vi "create.AddOrderLong.vi"(8 "error in (no error)":errorcluster, 10 "AddOrder.Parms":T1, 11 "AddOrderLong in":refnum<class "AddOrderLong.lvclass">) -> (0 "error out":errorcluster, 3 "AddOrderLong out":refnum<class "AddOrderLong.lvclass">)   [LabVIEW 2022 SP3, in "AddOrderLong.lvclass"]
uses:
  AddOrderLong.lvclass
  FieldSpec.ctl
  PitchMessage/FieldValue.ctl
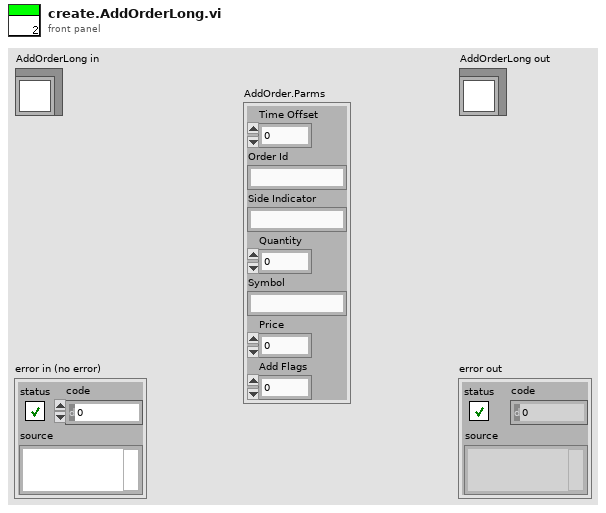
[diagram p1: front panel]
types:
  T1 = cluster{"Time Offset":u32, "Order Id":string, "Side Indicator":string, "Quantity":u32, "Symbol":string, "Price":dbl, "Add Flags":u8}
  T2 = typedef "FieldSpec.ctl" = cluster{"Name":string, "Offset":i32, "Length":i32, "FieldType":enum16{"Alphanumeric", "Binary", "BinaryLongPrice", "BinaryShortPrice", "BitField", "PrintableAscii", "Value"}}
  T3 = typedef "FieldValue.ctl" = variant
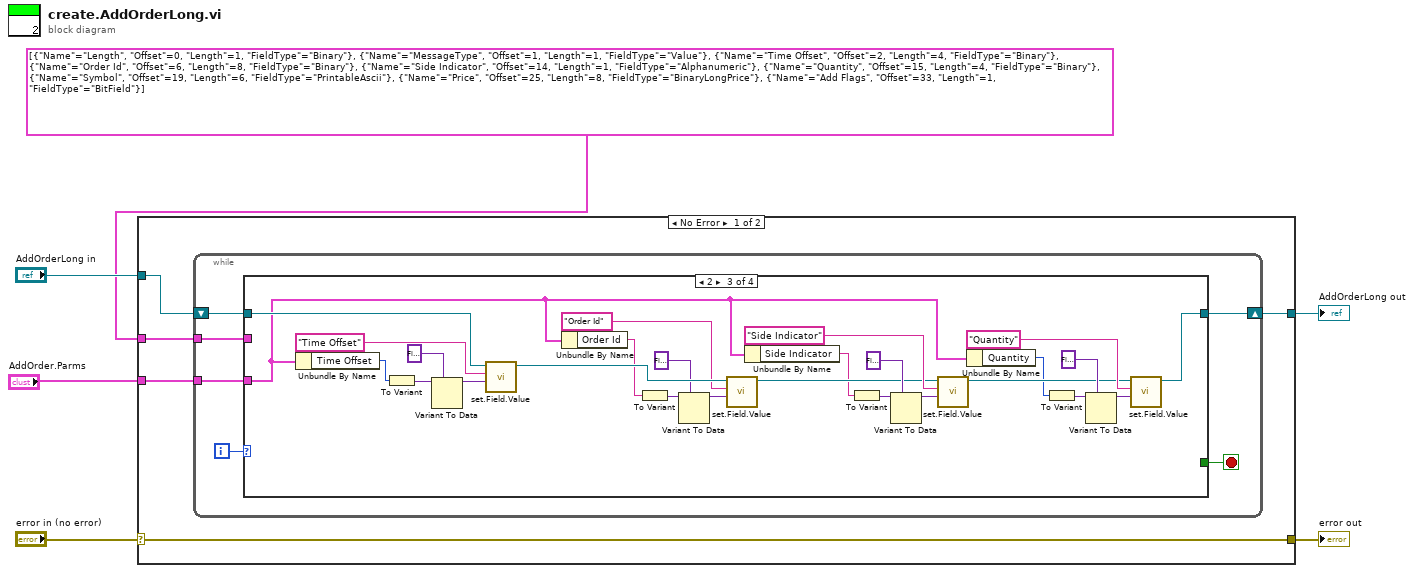
[diagram p0: block diagram]
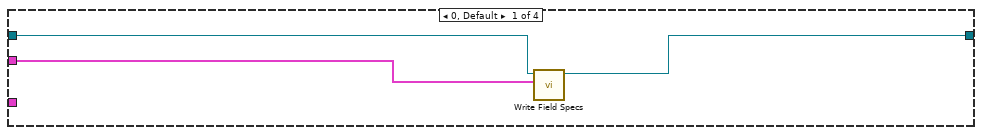
[diagram p2: hidden frame]
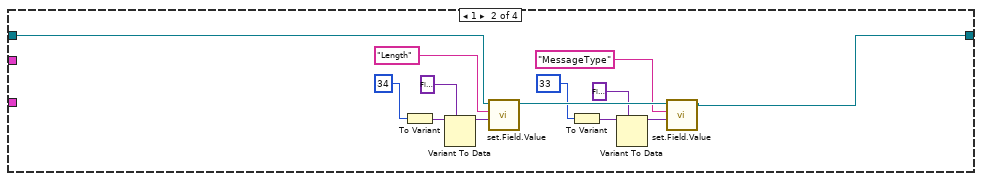
[diagram p3: hidden frame]
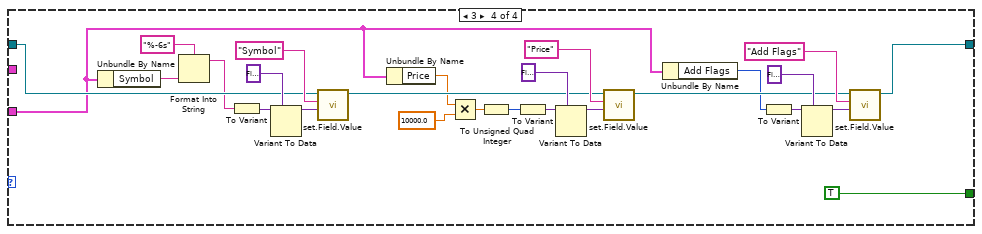
[diagram p4: hidden frame]
diagram:
  n1 = case shown="No Error" "error in (no error)" {
    selector: "error in (no error)" -> [w11 w87]
    tunnel: [w11 w87] -> w5
    tunnel: [w8 w86] -> w3
    tunnel: "AddOrderLong in" -> [w9 w86]
    tunnel: T2[] [{"Name"="Length", "Offset"=0, "Length"=1, "FieldType"=enum."Binary"}, {"Name"="MessageType", "Offset"=1, "Length"=1, "FieldType"=enum."Value"}, {"Name"="Time Offset", "Offset"=2, "Length"=4, "FieldType"=enum."Binary"}, {"Name"="Order Id", "Offset"=6, "Length"=8, "FieldType"=enum."Binary"}, {"Name"="Side Indicator", "Offset"=14, "Length"=1, "FieldType"=enum."Alphanumeric"}, {"Name"="Quantity", "Offset"=15, "Length"=4, "FieldType"=enum."Binary"}, {"Name"="Symbol", "Offset"=19, "Length"=6, "FieldType"=enum."PrintableAscii"}, {"Name"="Price", "Offset"=25, "Length"=8, "FieldType"=enum."BinaryLongPrice"}, {"Name"="Add Flags", "Offset"=33, "Length"=1, "FieldType"=enum."BitField"}] ("appended array") -> [w10 _]
    tunnel: "AddOrder.Parms" -> [w7 _]
    frame No Error {
      n2 = while {
        tunnel: w10 -> [w16]
        shift-right: [w14] -> w8
        shift-left: w9 -> [w15]
        tunnel: w7 -> [w12]
        i -> [w17]
        stop <- w13 stop-if-true
        n3 = case shown="2" w17 {
          tunnel: [_ _ _ TRUE] -> w13
          tunnel: w16 -> [w20 _ _ _]
          tunnel: w15 -> [w19 w22 w50 w81]
          tunnel: [w18 w21 w39 w64] -> w14
          tunnel: w12 -> [_ _ w35 w61]
          frame 0, Default {
            n4 = call-dynamic "Write Field Specs.vi"("Field Specs"=w20, "PitchMessage in"=w19) -> ("PitchMessage out"=w18:refnum<class "AddOrderLong.lvclass">)  [unwired: 8 in, 1 out]
          }
          frame 1 {
            n5 = To Variant(anything=u8 34 ("Value")) -> (Variant=w29:variant)
            n6 = Variant To Data(type=T3 variant ("FieldValue"), Variant=w29) -> (data=w30:T3)  [unwired: 1 in, 1 out]
            n7 = call-dynamic "set.Field.Value.vi"("Value"=w30, "FIeld.Name"="Length", "PitchMessage in"=w22) -> ("PitchMessage out"=w31:refnum<class "AddOrderLong.lvclass">)  [unwired: 7 in, 1 out]
            n8 = To Variant(anything=u8 33 ("Value")) -> (Variant=w32:variant)
            n9 = Variant To Data(type=T3 variant ("FieldValue"), Variant=w32) -> (data=w33:T3)  [unwired: 1 in, 1 out]
            n10 = call-dynamic "set.Field.Value.vi"("Value"=w33, "FIeld.Name"="MessageType", "PitchMessage in"=w31) -> ("PitchMessage out"=w21:refnum<class "AddOrderLong.lvclass">)  [unwired: 7 in, 1 out]
          }
          frame 2 {
            n11 = Unbundle By Name(w35) -> ("Time Offset"=w38:u32)
            n12 = To Variant(anything=w38) -> (Variant=w55:variant)
            n13 = Variant To Data(type=T3 variant ("FieldValue"), Variant=w55) -> (data=w56:T3)  [unwired: 1 in, 1 out]
            n14 = call-dynamic "set.Field.Value.vi"("Value"=w56, "FIeld.Name"="Time Offset", "PitchMessage in"=w50) -> ("PitchMessage out"=w58:refnum<class "AddOrderLong.lvclass">)  [unwired: 7 in, 1 out]
            n15 = Unbundle By Name(w35) -> ("Order Id"=w37:string)
            n16 = To Variant(anything=w37) -> (Variant=w57:variant)
            n17 = Variant To Data(type=T3 variant ("FieldValue"), Variant=w57) -> (data=w59:T3)  [unwired: 1 in, 1 out]
            n18 = call-dynamic "set.Field.Value.vi"("Value"=w59, "FIeld.Name"="Order Id", "PitchMessage in"=w58) -> ("PitchMessage out"=w45:refnum<class "AddOrderLong.lvclass">)  [unwired: 7 in, 1 out]
            n19 = Unbundle By Name(w35) -> ("Side Indicator"=w36:string)
            n20 = To Variant(anything=w36) -> (Variant=w48:variant)
            n21 = Variant To Data(type=T3 variant ("FieldValue"), Variant=w48) -> (data=w49:T3)  [unwired: 1 in, 1 out]
            n22 = call-dynamic "set.Field.Value.vi"("Value"=w49, "FIeld.Name"="Side Indicator", "PitchMessage in"=w45) -> ("PitchMessage out"=w40:refnum<class "AddOrderLong.lvclass">)  [unwired: 7 in, 1 out]
            n23 = Unbundle By Name(w35) -> ("Quantity"=w34:u32)
            n24 = To Variant(anything=w34) -> (Variant=w43:variant)
            n25 = Variant To Data(type=T3 variant ("FieldValue"), Variant=w43) -> (data=w44:T3)  [unwired: 1 in, 1 out]
            n26 = call-dynamic "set.Field.Value.vi"("Value"=w44, "FIeld.Name"="Quantity", "PitchMessage in"=w40) -> ("PitchMessage out"=w39:refnum<class "AddOrderLong.lvclass">)  [unwired: 7 in, 1 out]
          }
          frame 3 {
            n27 = Unbundle By Name(w61) -> ("Symbol"=w63:string)
            n28 = Format Into String(format string="%-6s", w63) -> (resulting string=w78:string)  [unwired: 2 in, 1 out]
            n29 = To Variant(anything=w78) -> (Variant=w84:variant)
            n30 = Variant To Data(type=T3 variant ("FieldValue"), Variant=w84) -> (data=w85:T3)  [unwired: 1 in, 1 out]
            n31 = call-dynamic "set.Field.Value.vi"("Value"=w85, "FIeld.Name"="Symbol", "PitchMessage in"=w81) -> ("PitchMessage out"=w70:refnum<class "AddOrderLong.lvclass">)  [unwired: 7 in, 1 out]
            n32 = Unbundle By Name(w61) -> ("Price"=w62:dbl)
            n33 = Multiply(x=w62, y=10000.0) -> (x*y=w72:dbl)
            n34 = To Unsigned Quad Integer(1:w72) -> (0:w71:u64)
            n35 = To Variant(anything=w71) -> (Variant=w76:variant)
            n36 = Variant To Data(type=T3 variant ("FieldValue"), Variant=w76) -> (data=w77:T3)  [unwired: 1 in, 1 out]
            n37 = call-dynamic "set.Field.Value.vi"("Value"=w77, "FIeld.Name"="Price", "PitchMessage in"=w70) -> ("PitchMessage out"=w65:refnum<class "AddOrderLong.lvclass">)  [unwired: 7 in, 1 out]
            n38 = Unbundle By Name(w61) -> ("Add Flags"=w60:u8)
            n39 = To Variant(anything=w60) -> (Variant=w68:variant)
            n40 = Variant To Data(type=T3 variant ("FieldValue"), Variant=w68) -> (data=w69:T3)  [unwired: 1 in, 1 out]
            n41 = call-dynamic "set.Field.Value.vi"("Value"=w69, "FIeld.Name"="Add Flags", "PitchMessage in"=w65) -> ("PitchMessage out"=w64:refnum<class "AddOrderLong.lvclass">)  [unwired: 7 in, 1 out]
          }
        }
      }
    }
    frame Error {
    }
  }
  "error out" <- w5
  "AddOrderLong out" <- w3
